vi "Poll.Initialize.vi"(7 "FirstCall?":bool, 8 "error in (no error)":errorcluster, 10 "Parameters in":T2 {"Settings"."Data Refs"."Write Refs" format="%.0x"; "Settings"."Data Refs"."Read Refs" format="%.0x"; "Settings"."Write Locations"."DataType" items=["Boolean"=1, "SByte"=2, "Byte"=3, "Int16"=4, "UInt16"=5, "Int32"=6, "UInt32"=7, "Int64"=8, "UInt64"=9, "Float"=10, "Double"=11, "String"=12, "DateTime"=13, "ByteString"=15, "Array of Boolean"=101, "Array of SByte"=102, "Array of Byte"=103, "Array of Int16"=104, "Array of UInt16"=105, "Array of Int32"=106, "Array of UInt32"=107, "Array of Int64"=108, "Array of UInt64"=109, "Array of Float"=110, "Array of Double"=111, "Array of String"=112, "Array of DateTime"=113, "Array of ByteString"=115]}, 11 "Process":refnum<class "Process.lvclass">) -> (0 "error out":errorcluster, 1 "notification":bool, 2 "Parameters out":T2 {"Settings"."Data Refs"."Write Refs" format="%.0x"; "Settings"."Data Refs"."Read Refs" format="%.0x"; "Settings"."Write Locations"."DataType" items=["Boolean"=1, "SByte"=2, "Byte"=3, "Int16"=4, "UInt16"=5, "Int32"=6, "UInt32"=7, "Int64"=8, "UInt64"=9, "Float"=10, "Double"=11, "String"=12, "DateTime"=13, "ByteString"=15, "Array of Boolean"=101, "Array of SByte"=102, "Array of Byte"=103, "Array of Int16"=104, "Array of UInt16"=105, "Array of Int32"=106, "Array of UInt32"=107, "Array of Int64"=108, "Array of UInt64"=109, "Array of Float"=110, "Array of Double"=111, "Array of String"=112, "Array of DateTime"=113, "Array of ByteString"=115]}, 3 "Settings":T1)   [LabVIEW 2015, in "OPC UA Client Engine.lvlib"]
uses:
  OPC UA Client Engine.lvlib
  Types/Poll.Parameters.ctl
  Shared/Compiled.Settings.ctl
  Shared/OPCConnection.Properties.ctl
  Shared/Poll.ListProperties.ctl
  Shared/Tag.WriteProperties.Info.ctl
  Shared/Tags.ReadWriteRefs.ctl
  <vilib>/NI Veristand/Custom Device API/Data Reference.ctl
  <vilib>/NI Veristand/Custom Device API/Custom Device Target Type.ctl
  Types/Poll.StateVariables.ctl
  <vilib>/NI/NI VeriStand Inline Async API/_VS Inline Async API/Process/Process.lvclass
  <vilib>/NI/NI VeriStand Inline Async API/_Data Access Engine/Access Type Classes/Write/Write.lvclass
  <vilib>/NI/NI VeriStand Inline Async API/_VS Inline Async API/Process/Process.lvclass/Process.ctl
  <vilib>/NI/NI VeriStand Inline Async API/_VS Inline Async API/Process/Data Member Access/Read Data Access.vi
  <vilib>/NI/NI VeriStand Inline Async API/_VS Inline Async API/Error Handling Process/SubVIs/Error.ConvertArray.vi
  <vilib>/NI/NI VeriStand Inline Async API/_Data Access Engine/Data Access Engine/Methods/Write.Lookup.vi
  Shared/Constants.vi
  <vilib>/NI/NI VeriStand Inline Async API/_Data Access Engine/Data Access Engine/Data Access Engine.lvclass
  <vilib>/OPCUA/NI OPC UA Client.lvlib
  Stop FG/Stop FG.lvlib
  <vilib>/NI Veristand/Custom Device Tools/Custom Device Utility Library/Custom Device Utility Library.lvlib
  Shared/OPC UA Client Shared.lvlib
  <vilib>/NI VeriStand/Custom Device API/Custom Device API.lvlib
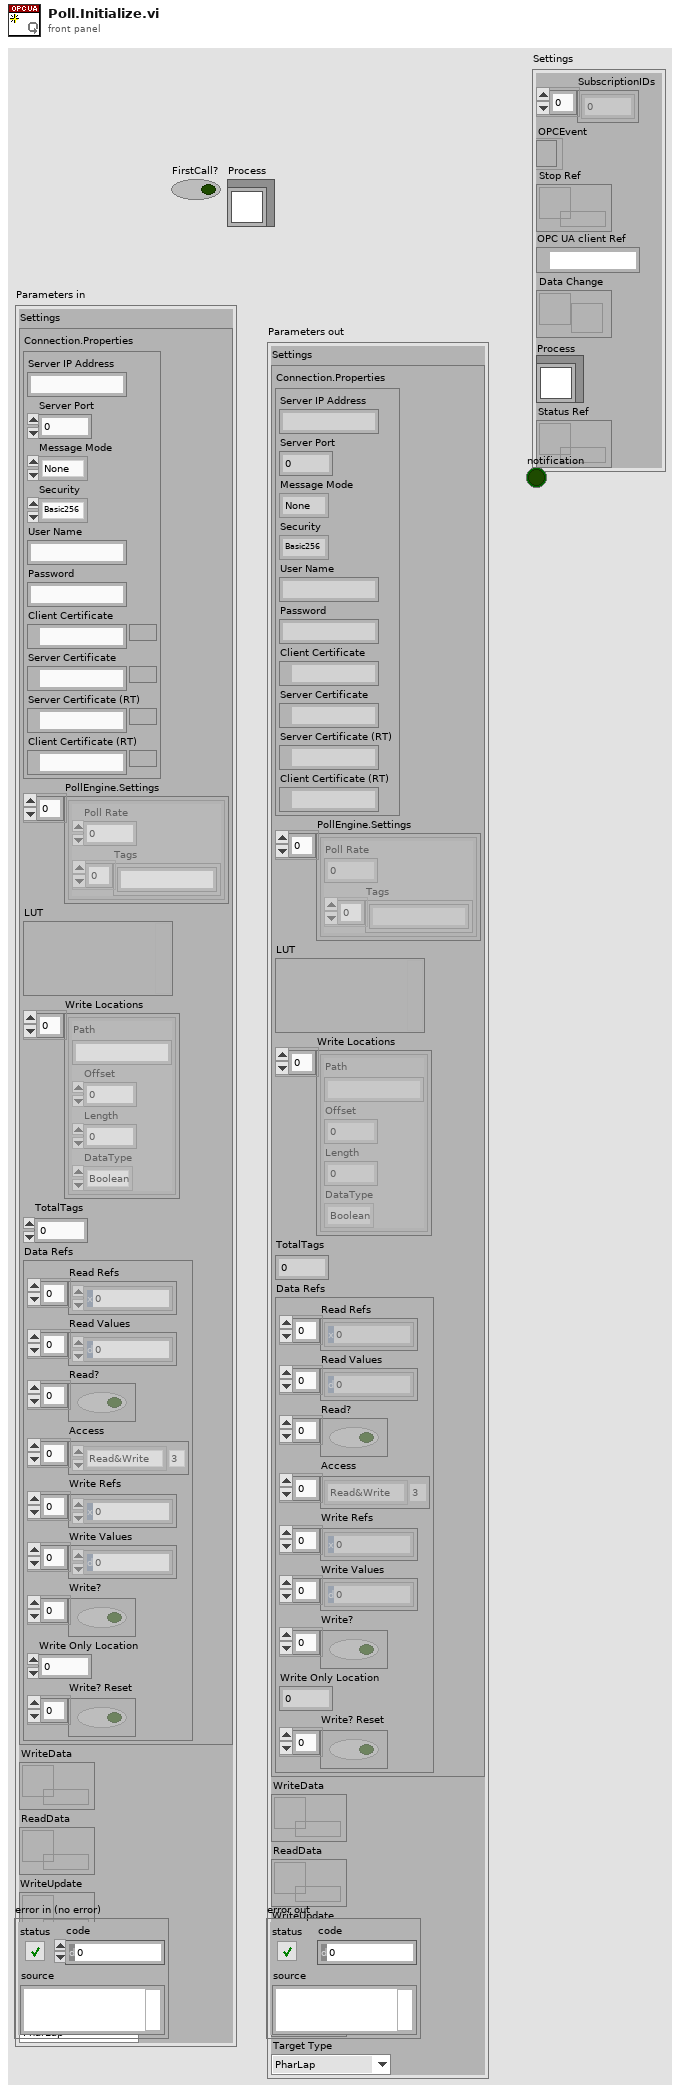
[diagram p1: front panel]
types:
  T1 = typedef "OPC UA Client Engine.lvlib/Poll.StateVariables.ctl" = cluster{"SubscriptionIDs":u32[], "OPCEvent":refnum<event-registration>, "Stop Ref":refnum<data-value>, "OPC UA client Ref":refnum<k21>, "Data Change":refnum<user-event>, "Process":refnum<class "Process.lvclass">, "Status Ref":refnum<data-value>}
  T2 = typedef "OPC UA Client Engine.lvlib/Poll.Parameters.ctl" = cluster{"Settings":T3, "WriteData":refnum<k33>, "ReadData":refnum<k33>, "WriteUpdate":refnum<k33>, "ReadUpdate":refnum<k33>, "Target Type":T9}
  T3 = typedef "OPC UA Client Shared.lvlib/Compiled.Settings.ctl" = cluster{"Connection.Properties":T4, "PollEngine.Settings":T5[], "LUT":variant, "Write Locations":T6[], "TotalTags":u32, "Data Refs":T7}
  T4 = typedef "OPC UA Client Shared.lvlib/OPCConnection.Properties.ctl" = cluster{"Server IP Address":string, "Server Port":u16, "Message Mode":enum16{"None", "Sign", "Sign and Encrypt"}, "Security":enum16{"Basic256", "Basic128Rsa15"}, "User Name":string, "Password":string, "Client Certificate":path, "Server Certificate":path, "Server Certificate (RT)":path, "Client Certificate (RT)":path}
  T5 = typedef "OPC UA Client Shared.lvlib/Poll.ListProperties.ctl" = cluster{"Poll Rate":dbl, "Tags":string[]}
  T6 = typedef "OPC UA Client Shared.lvlib/Tag.WriteProperties.Info.ctl" = cluster{"Path":string, "Offset":i32, "Length":i32, "DataType":u32}
  T7 = typedef "OPC UA Client Shared.lvlib/Tags.ReadWriteRefs.ctl" = cluster{"Read Refs":T8[], "Read Values":dbl[], "Read?":bool[], "Access":enum8{"Null", "Read", "Write", "Read&Write"}[], "Write Refs":T8[], "Write Values":dbl[], "Write?":bool[], "Write Only Location":u32, "Write? Reset":bool[]}
  T8 = typedef "Custom Device API.lvlib/Data Reference.ctl" = i32
  T9 = typedef "Custom Device API.lvlib/Custom Device Target Type.ctl" = enum16{"PharLap", "VxWorks", "Windows", "Linux_32_ARM", "Linux_x64"}
  T10 = cluster{"message mode":enum16{"None", "Sign", "Sign and Encrypt"}, "security":enum16{"Basic256", "Basic128Rsa15"}}
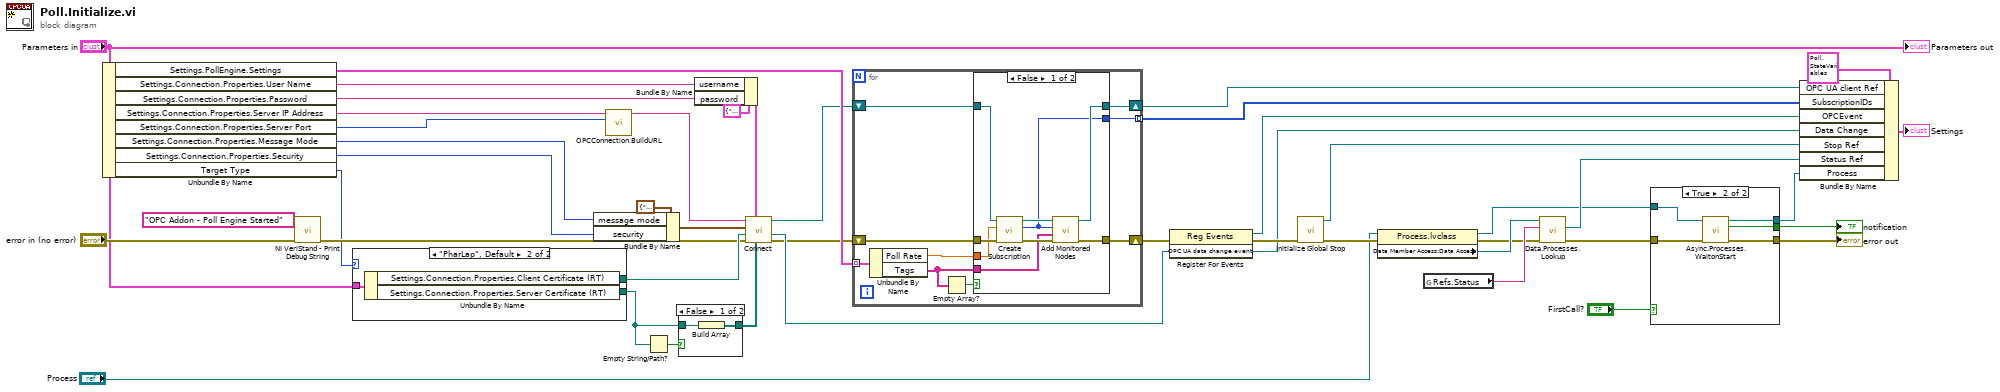
[diagram p0: block diagram]
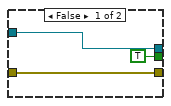
[diagram p2: hidden frame]
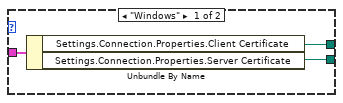
[diagram p4: hidden frame]
diagram:
  n1 = Unbundle By Name("Parameters in") -> ("Settings.PollEngine.Settings"=w18:T5[], "Settings.Connection.Properties.User Name"=w25:string, "Settings.Connection.Properties.Password"=w24:string, "Settings.Connection.Properties.Server IP Address"=w30:string, "Settings.Connection.Properties.Server Port"=w29:u16, "Settings.Connection.Properties.Message Mode"=w23:enum16{"None", "Sign", "Sign and Encrypt"}, "Settings.Connection.Properties.Security"=w22:enum16{"Basic256", "Basic128Rsa15"}, "Target Type"=w17:T9)
  n2 = call <vilib>:"NI VeriStand - Print Debug String.vi"("error in (no error)"="error in (no error)", "Message"="OPC Addon - Poll Engine Started") -> ("error out"=w19:errorcluster)  [unwired: 9 in]
  n3 = case shown="\"PharLap\", Default" w17 {
    tunnel: [w47 w50] -> w21
    tunnel: [w46 w49] -> w28
    tunnel: "Parameters in" -> [w45 w48]
    frame "Windows" {
      n4 = Unbundle By Name(w45) -> ("Settings.Connection.Properties.Client Certificate"=w47:path, "Settings.Connection.Properties.Server Certificate"=w46:path)
    }
    frame "PharLap", Default {
      n5 = Unbundle By Name(w48) -> ("Settings.Connection.Properties.Client Certificate (RT)"=w50:path, "Settings.Connection.Properties.Server Certificate (RT)"=w49:path)
    }
  }
  n6 = Bundle By Name(cluster=T10 {"message mode"=enum."Sign", "security"=enum."Basic256"} ("security policy"), "message mode"=w23, "security"=w22) -> (w31:T10)
  n7 = call "OPCConnection.BuildURL.vi"("Server Port"=w29, "Server IP Address"=w30) -> ("OPC Path"=w26:string)  [unwired: 9 in]
  n8 = Empty String/Path?(string/path=w28) -> (empty?=w20:bool)
  n9 = case shown="False" w20 {
    tunnel: [w52 _] -> w27
    tunnel: w28 -> [w51 _]
    frame False {
      n10 = Build Array(w51) -> (w52:path[])
    }
    frame True {
    }
  }
  n11 = Bundle By Name(cluster=cluster{"username":string, "password":string} {"username"="", "password"=""} ("username/password"), "username"=w25, "password"=w24) -> (w33:cluster{"username":string, "password":string})
  n12 = call <vilib>:"Connect.vi"("trusted server certificates"=w27, "username/password"=w33, "error in (no error)"=w19, "client certificate file"=w21, "security policy"=w31, "server endpoint URL"=w26) -> ("error out"=w12:errorcluster, "OPC UA data change event"=w15:refnum<user-event>, "OPC UA client refnum out"=w16:refnum<k21>)  [unwired: 3 in]
  n13 = for {
    tunnel: [w59] -> w42 mode=indexing
    tunnel: w18 -> [w56] mode=indexing
    shift-right: [w60] -> w11
    shift-left: w12 -> [w57]
    shift-right: [w61] -> w13
    shift-left: w16 -> [w58]
    n14 = Unbundle By Name(w56) -> ("Poll Rate"=w55:dbl, "Tags"=w53:string[])
    n15 = Empty Array?(array=w53) -> (empty?=w54:bool)
    n16 = case shown="False" w54 {
      tunnel: [w68 w72] -> w61
      tunnel: [w67 w71] -> w60
      tunnel: [w66 _] -> w59
      tunnel: w58 -> [w65 w72]
      tunnel: w57 -> [w64 w71]
      tunnel: w55 -> [w63 _]
      tunnel: w53 -> [w62 _]
      frame False {
        n17 = call <vilib>:"Create Subscription.vi"("error in (no error)"=w64, "update rate (1000 ms)"=w63, "OPC UA client refnum in"=w65) -> ("error out"=w69:errorcluster, "subscription ID out"=w66:u32, "OPC UA client refnum out"=w70:refnum<k21>)  [unwired: 6 in]
        n18 = call <vilib>:"Add Monitored Nodes.vi"("error in (no error)"=w69, "array of node path"=w62, "subscription ID in"=w66, "OPC UA client refnum in"=w70) -> ("error out"=w67:errorcluster, "OPC UA client refnum out"=w68:refnum<k21>)  [unwired: 5 in, 1 out]
      }
      frame True {
      }
    }
  }
  n19 = register-events(error in=w11, w15) -> (reference out=w40:refnum<event-registration>, error out=w43:errorcluster)  [unwired: 1 in]
  n20 = call "Initialize Global Stop.vi"("error in (no error)"=w43) -> ("error out"=w5:errorcluster, "Stop Ref"=w41:refnum<data-value>)  [unwired: 9 in]
  n21 = property class="Process.lvclass"(reference="Process", error in=w5) -> (reference out=w1:refnum<class "Process.lvclass">, error out=w4:errorcluster, "Data Member Access:Data Access"=w8:refnum<class "Data Access Engine.lvclass">)
  n22 = global read "Constants.vi" "Refs.Status"() -> (w7:string)
  n23 = call-poly <vilib>:"Data.Processes.Lookup.vi"("error in (no error)"=w4, "Name"=w7, "Data Access API in"=w8) -> ("error out"=w6:errorcluster, "Ref"=w3:refnum<data-value>)  [unwired: 5 in, 2 out]
  n24 = case shown="True" "FirstCall?" {
    tunnel: [w75 w78] -> w44
    tunnel: [TRUE ("notification") w77] -> w37
    tunnel: w6 -> [w75 w79]
    tunnel: w1 -> [w73 w80]
    tunnel: [w73 w76] -> w9
    frame False {
    }
    frame True {
      n25 = call <vilib>:"Async.Processes.WaitonStart.vi"("error in (no error)"=w79, "Process"=w80) -> ("error out"=w78:errorcluster, "Execute"=w77:bool, "Process out"=w76:refnum<class "Process.lvclass">)  [unwired: 7 in]
    }
  }
  "error out" <- w44
  "notification" <- w37
  n26 = Bundle By Name(cluster=T1 {"SubscriptionIDs"=[], "OPCEvent"=refnum, "Stop Ref"=refnum, "OPC UA client Ref"="", "Data Change"=refnum, "Process"=refnum, "Status Ref"=refnum} ("output cluster"), "OPC UA client Ref"=w13, "SubscriptionIDs"=w42, "OPCEvent"=w40, "Data Change"=w15, "Stop Ref"=w41, "Status Ref"=w3, "Process"=w9) -> (→"Settings":T1)
  "Parameters out" <- "Parameters in"
